vi "Rapid Read_5Ch.vi"(0 "Dig Cards":refnum<k15>[](array[refnum]), 2 "Pause?":bool, 5 "Motion Board ID":T1=1 min=1 max=32 step=1, 9 "rf points per line":i32, 11 "error in":errorcluster, 12 "lines per plane":i32, 13 "queue out":refnum<queue>) -> (1 "gain":dbl, 6 "Reverse?":bool, 10 "Dig Word Size":u16, 15 "error out":errorcluster)   [LabVIEW 2022 SP3]
uses:
  Motion Controllers/-MotionRoutines/MotionGlobals.vi
  <instrlib>/niScope/Acquire/Fetch/niScope Multi Fetch Binary 8.vi
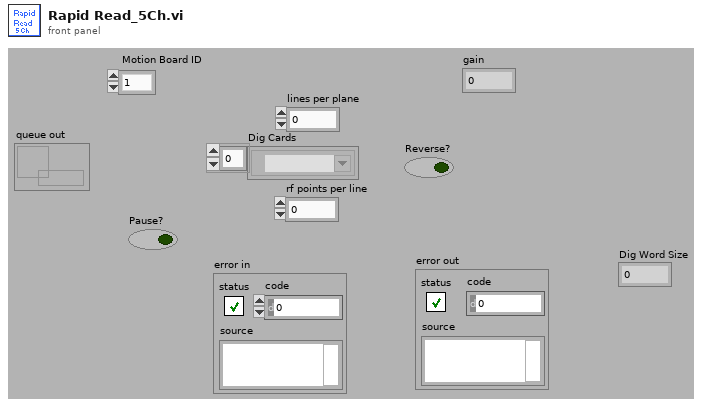
[diagram p1: front panel]
types:
  T1 = typedef "Board Id" = u8
  T2 = cluster{"Dig Cards[0]":refnum<k15>, "Dig Cards[1]":refnum<k15>, "Dig Cards[2]":refnum<k15>}
  T3 = typedef "Var" = u8
  T4 = cluster{"actualSamples":i32, "absoluteInitialX":dbl, "relativeInitialX":dbl, "xIncrement":dbl, "offset":dbl, "gain":dbl, "reserved1":dbl, "reserved2":dbl}[]
  T5 = cluster{"actualSamples":i32, "absoluteInitialX":dbl, "relativeInitialX":dbl, "xIncrement":dbl, "offset":dbl, "gain":dbl, "reserved1":dbl, "reserved2":dbl}
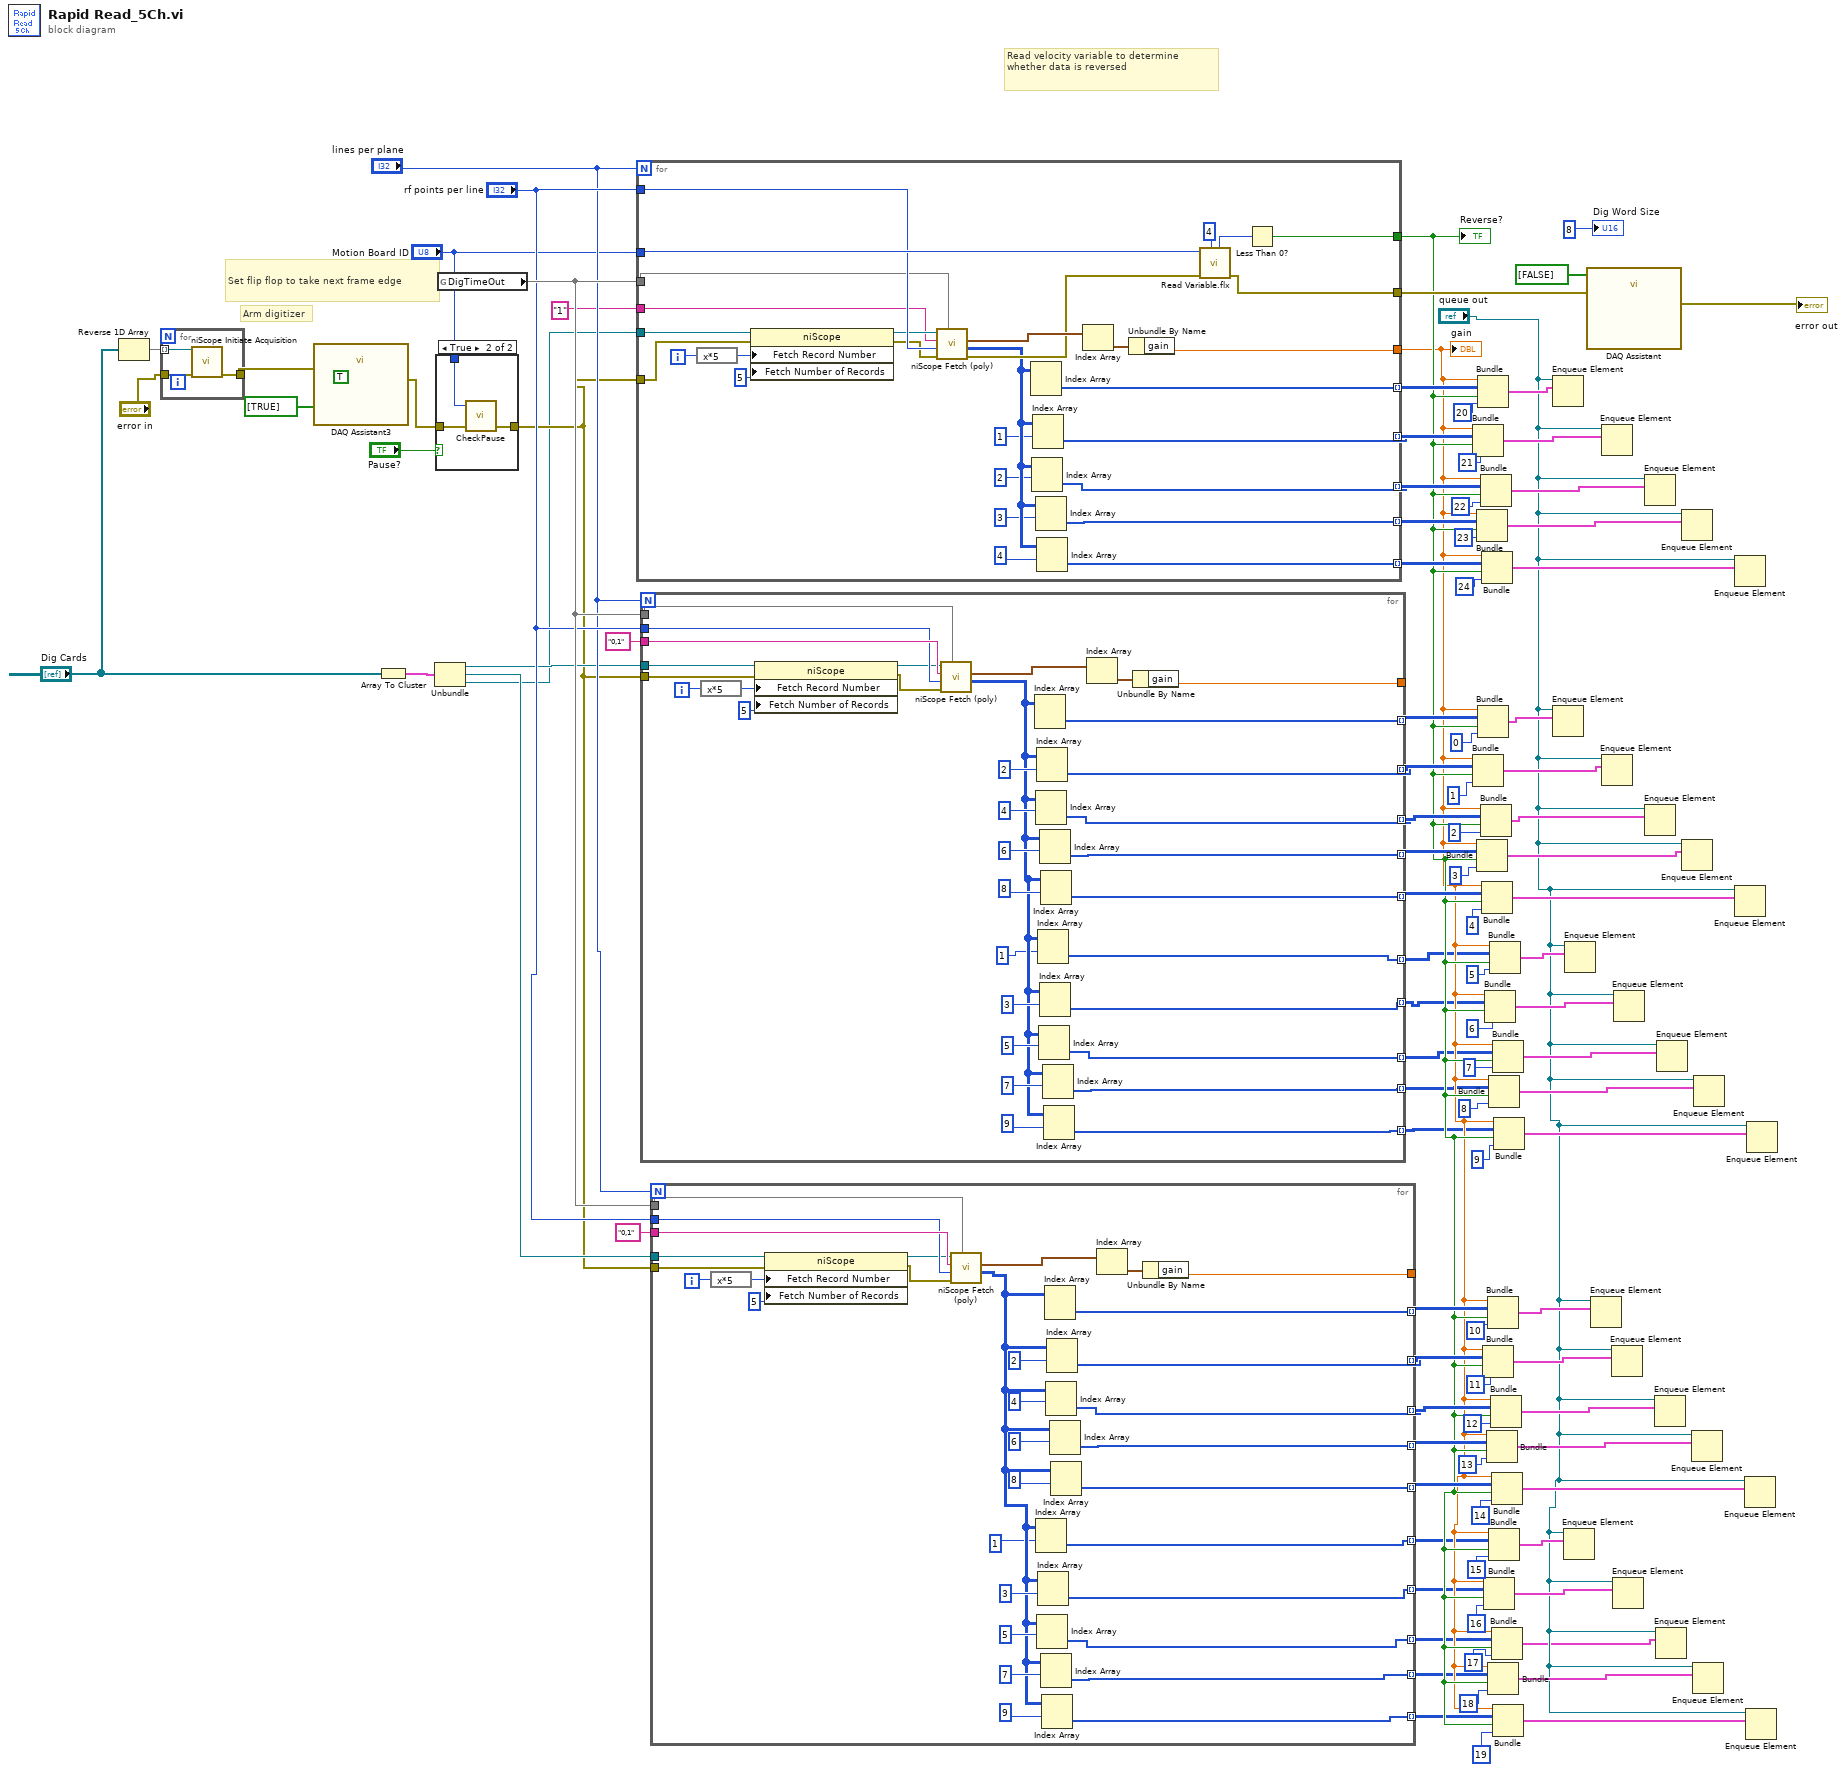
[diagram p0: block diagram]
diagram:
  (unwired) TRUE ("stop (T)")
  # "Set flip flop to take next frame edge"
  # "Arm digitizer"
  # "Read velocity variable to determine whether data is reversed"
  n1 = Reverse 1D Array(array="Dig Cards") -> (reversed array=w37:refnum<k15>[])
  n2 = for {
    tunnel: w37 -> [w104] mode=indexing
    tunnel: [w103] -> w36
    tunnel: "error in" -> [w102]
    n3 = call <instrlib>:"niScope Initiate Acquisition.vi"("instrument handle"=w104, "error in"=w102) -> ("error out"=w103:errorcluster)  [unwired: 1 in, 12 out]
  }
  n4 = call "DAQ Assistant3"("data"=bool[] [TRUE], "error in"=w36) -> ("error out"=w42:errorcluster)  [unwired: 2 in, 15 out]
  n5 = Array To Cluster(array="Dig Cards") -> (cluster=w97:T2)
  n6 = Unbundle(w97) -> ("Dig Cards[0]"=w44:refnum<k15>, "Dig Cards[1]"=w43:refnum<k15>, "Dig Cards[2]"=w35:refnum<k15>)
  n7 = case shown="True" "Pause?" {
    tunnel: w42 -> [w105 w108]
    tunnel: [w105 w107] -> w41
    tunnel: "Motion Board ID" -> [_ w106]
    frame False {
    }
    frame True {
      n8 = call "CheckPause.vi"("error in"=w108, "Motion Board ID"=w106) -> ("error out"=w107:errorcluster)  [unwired: 3 in]
    }
  }
  n9 = global read "MotionGlobals.vi" "DigTimeOut"() -> (w58)
  n10 = for {
    N: "lines per plane" -> [_]
    tunnel: "Motion Board ID" -> [w137]
    tunnel: "rf points per line" -> [w136]
    tunnel: w58 -> [w135]
    tunnel: w35 -> [w134]
    tunnel: w41 -> [w133]
    tunnel: "1" ("Channel") -> [w125]
    tunnel: [w119] -> w96 mode=indexing
    tunnel: [w118] -> w95 mode=indexing
    tunnel: [w117] -> w94 mode=indexing
    tunnel: [w116] -> w93 mode=indexing
    tunnel: [w115] -> w92 mode=indexing
    tunnel: [w111] -> w60
    tunnel: [w110] -> w59
    tunnel: [w109] -> w87
    i -> [w126]
    n11 = expression code="x*5"(w126) -> (w127:i32)
    n12 = property class="niScope"(reference=w134, error in=w133, "Fetch Record Number"=w127, "Fetch Number of Records"=5) -> (reference out=w132:refnum<k15>, error out=w131:errorcluster)
    n13 = call-poly <instrlib>:"niScope Fetch (poly).vi"("timeout"=w135, "error in"=w131, "numSamples"=w136, "channels"=w125, "instrument handle"=w132) -> ("error out"=w129:errorcluster, "wfm"=w124:i8[][], "wfm info"=w130:T4)  [unwired: 4 out]
    n14 = Index Array(array=w124) -> (element=w119:i8[])  [unwired: 2 in]
    n15 = Index Array(array=w124, index (row)=2) -> (element=w117:i8[])  [unwired: 1 in]
    n16 = Index Array(array=w124, index (row)=1) -> (element=w118:i8[])  [unwired: 1 in]
    n17 = Index Array(array=w124, index (row)=3) -> (element=w116:i8[])  [unwired: 1 in]
    n18 = Index Array(array=w124, index (row)=4) -> (element=w115:i8[])  [unwired: 1 in]
    n19 = Index Array(array=w130) -> (element=w112:T5)  [unwired: 1 in]
    n20 = Unbundle By Name(w112) -> ("gain"=w110:dbl)
    n21 = call <vilib>:"Read Variable.flx"("Var"=T3 4, "error in (no error)"=w129, "Board ID"=w137) -> ("error out"=w109:errorcluster, "Output"=w113:i32)  [unwired: 1 in, 4 out]
    n22 = Less Than 0?(x=w113) -> (x < 0?=w111:bool)
  }
  "Reverse?" <- w60
  "gain" <- w59
  n23 = for {
    N: "lines per plane" -> [_]
    tunnel: "rf points per line" -> [w150]
    tunnel: w58 -> [w148]
    tunnel: w44 -> [w170]
    tunnel: "0,1" ("Channel") -> [w165]
    tunnel: [w161] -> w85 mode=indexing
    tunnel: [w160] -> w84 mode=indexing
    tunnel: [w159] -> w83 mode=indexing
    tunnel: [w158] -> w82 mode=indexing
    tunnel: [w157] -> w81 mode=indexing
    tunnel: [w155] -> _
    tunnel: [w146] -> w55 mode=indexing
    tunnel: [w145] -> w54 mode=indexing
    tunnel: [w144] -> w53 mode=indexing
    tunnel: [w143] -> w52 mode=indexing
    tunnel: [w142] -> w51 mode=indexing
    tunnel: w41 -> [w141]
    i -> [w166]
    n24 = expression code="x*5"(w166) -> (w167:i32)
    n25 = property class="niScope"(reference=w170, error in=w141, "Fetch Record Number"=w167, "Fetch Number of Records"=5) -> (reference out=w149:refnum<k15>, error out=w147:errorcluster)
    n26 = call-poly <instrlib>:"niScope Fetch (poly).vi"("timeout"=w148, "error in"=w147, "numSamples"=w150, "channels"=w165, "instrument handle"=w149) -> ("wfm"=w139:i8[][], "wfm info"=w169:T4)  [unwired: 5 out]
    n27 = Index Array(array=w139) -> (element=w161:i8[])  [unwired: 2 in]
    n28 = Index Array(array=w139, index (row)=4) -> (element=w159:i8[])  [unwired: 1 in]
    n29 = Index Array(array=w139, index (row)=2) -> (element=w160:i8[])  [unwired: 1 in]
    n30 = Index Array(array=w139, index (row)=1) -> (element=w146:i8[])  [unwired: 1 in]
    n31 = Index Array(array=w139, index (row)=5) -> (element=w144:i8[])  [unwired: 1 in]
    n32 = Index Array(array=w139, index (row)=6) -> (element=w158:i8[])  [unwired: 1 in]
    n33 = Index Array(array=w139, index (row)=3) -> (element=w145:i8[])  [unwired: 1 in]
    n34 = Index Array(array=w139, index (row)=8) -> (element=w157:i8[])  [unwired: 1 in]
    n35 = Index Array(array=w139, index (row)=7) -> (element=w143:i8[])  [unwired: 1 in]
    n36 = Index Array(array=w139, index (row)=9) -> (element=w142:i8[])  [unwired: 1 in]
    n37 = Index Array(array=w169) -> (element=w156:T5)  [unwired: 1 in]
    n38 = Unbundle By Name(w156) -> ("gain"=w155:dbl)
  }
  n39 = for {
    N: "lines per plane" -> [_]
    tunnel: "rf points per line" -> [w182]
    tunnel: w58 -> [w181]
    tunnel: w43 -> [w203]
    tunnel: "0,1" ("Channel") -> [w198]
    tunnel: [w193] -> w69 mode=indexing
    tunnel: [w192] -> w68 mode=indexing
    tunnel: [w191] -> w67 mode=indexing
    tunnel: [w190] -> w66 mode=indexing
    tunnel: [w189] -> w65 mode=indexing
    tunnel: [w187] -> _
    tunnel: [w178] -> w50 mode=indexing
    tunnel: [w177] -> w49 mode=indexing
    tunnel: [w176] -> w48 mode=indexing
    tunnel: [w175] -> w47 mode=indexing
    tunnel: [w174] -> w46 mode=indexing
    tunnel: w41 -> [w173]
    i -> [w199]
    n40 = expression code="x*5"(w199) -> (w200:i32)
    n41 = property class="niScope"(reference=w203, error in=w173, "Fetch Record Number"=w200, "Fetch Number of Records"=5) -> (reference out=w180:refnum<k15>, error out=w179:errorcluster)
    n42 = call-poly <instrlib>:"niScope Fetch (poly).vi"("timeout"=w181, "error in"=w179, "numSamples"=w182, "channels"=w198, "instrument handle"=w180) -> ("wfm"=w172:i8[][], "wfm info"=w202:T4)  [unwired: 5 out]
    n43 = Index Array(array=w172, index (row)=1) -> (element=w178:i8[])  [unwired: 1 in]
    n44 = Index Array(array=w172, index (row)=5) -> (element=w176:i8[])  [unwired: 1 in]
    n45 = Index Array(array=w172, index (row)=3) -> (element=w177:i8[])  [unwired: 1 in]
    n46 = Index Array(array=w172, index (row)=7) -> (element=w175:i8[])  [unwired: 1 in]
    n47 = Index Array(array=w172, index (row)=9) -> (element=w174:i8[])  [unwired: 1 in]
    n48 = Index Array(array=w172) -> (element=w193:i8[])  [unwired: 2 in]
    n49 = Index Array(array=w172, index (row)=4) -> (element=w191:i8[])  [unwired: 1 in]
    n50 = Index Array(array=w172, index (row)=2) -> (element=w192:i8[])  [unwired: 1 in]
    n51 = Index Array(array=w172, index (row)=6) -> (element=w190:i8[])  [unwired: 1 in]
    n52 = Index Array(array=w172, index (row)=8) -> (element=w189:i8[])  [unwired: 1 in]
    n53 = Index Array(array=w202) -> (element=w188:T5)  [unwired: 1 in]
    n54 = Unbundle By Name(w188) -> ("gain"=w187:dbl)
  }
  n55 = Bundle("gain"=w59, "wfm"=w95, w60, 21) -> (w91:cluster{"gain":dbl, "wfm":i8[][], bool, i32})  [unwired: 1 in]
  n56 = Bundle("gain"=w59, "wfm"=w84, w60, 1) -> (w6:cluster{"gain":dbl, "wfm":i8[][], bool, i32})  [unwired: 1 in]
  n57 = Bundle("gain"=w59, "wfm"=w93, w60, 23) -> (w89:cluster{"gain":dbl, "wfm":i8[][], bool, i32})  [unwired: 1 in]
  n58 = Bundle("gain"=w59, "wfm"=w82, w60, 3) -> (w8:cluster{"gain":dbl, "wfm":i8[][], bool, i32})  [unwired: 1 in]
  n59 = Bundle("gain"=w59, "wfm"=w96, w60, 20) -> (w4:cluster{"gain":dbl, "wfm":i8[][], bool, i32})  [unwired: 1 in]
  n60 = Bundle("gain"=w59, "wfm"=w85, w60, 0) -> (w5:cluster{"gain":dbl, "wfm":i8[][], bool, i32})  [unwired: 1 in]
  n61 = Bundle("gain"=w59, "wfm"=w94, w60, 22) -> (w90:cluster{"gain":dbl, "wfm":i8[][], bool, i32})  [unwired: 1 in]
  n62 = Bundle("gain"=w59, "wfm"=w83, w60, 2) -> (w7:cluster{"gain":dbl, "wfm":i8[][], bool, i32})  [unwired: 1 in]
  n63 = Bundle("gain"=w59, "wfm"=w92, w60, 24) -> (w88:cluster{"gain":dbl, "wfm":i8[][], bool, i32})  [unwired: 1 in]
  n64 = Bundle("gain"=w59, "wfm"=w81, w60, 4) -> (w9:cluster{"gain":dbl, "wfm":i8[][], bool, i32})  [unwired: 1 in]
  n65 = Bundle("gain"=w59, "wfm"=w68, w60, 11) -> (w73:cluster{"gain":dbl, "wfm":i8[][], bool, i32})  [unwired: 1 in]
  n66 = Bundle("gain"=w59, "wfm"=w49, w60, 16) -> (w63:cluster{"gain":dbl, "wfm":i8[][], bool, i32})  [unwired: 1 in]
  n67 = Bundle("gain"=w59, "wfm"=w54, w60, 6) -> (w79:cluster{"gain":dbl, "wfm":i8[][], bool, i32})  [unwired: 1 in]
  n68 = Bundle("gain"=w59, "wfm"=w66, w60, 13) -> (w71:cluster{"gain":dbl, "wfm":i8[][], bool, i32})  [unwired: 1 in]
  n69 = Bundle("gain"=w59, "wfm"=w69, w60, 10) -> (w74:cluster{"gain":dbl, "wfm":i8[][], bool, i32})  [unwired: 1 in]
  n70 = Bundle("gain"=w59, "wfm"=w47, w60, 18) -> (w62:cluster{"gain":dbl, "wfm":i8[][], bool, i32})  [unwired: 1 in]
  n71 = Bundle("gain"=w59, "wfm"=w52, w60, 8) -> (w77:cluster{"gain":dbl, "wfm":i8[][], bool, i32})  [unwired: 1 in]
  n72 = Bundle("gain"=w59, "wfm"=w50, w60, 15) -> (w64:cluster{"gain":dbl, "wfm":i8[][], bool, i32})  [unwired: 1 in]
  n73 = Bundle("gain"=w59, "wfm"=w55, w60, 5) -> (w80:cluster{"gain":dbl, "wfm":i8[][], bool, i32})  [unwired: 1 in]
  n74 = Bundle("gain"=w59, "wfm"=w67, w60, 12) -> (w72:cluster{"gain":dbl, "wfm":i8[][], bool, i32})  [unwired: 1 in]
  n75 = Bundle("gain"=w59, "wfm"=w65, w60, 14) -> (w70:cluster{"gain":dbl, "wfm":i8[][], bool, i32})  [unwired: 1 in]
  n76 = Bundle("gain"=w59, "wfm"=w48, w60, 17) -> (w2:cluster{"gain":dbl, "wfm":i8[][], bool, i32})  [unwired: 1 in]
  n77 = Bundle("gain"=w59, "wfm"=w53, w60, 7) -> (w78:cluster{"gain":dbl, "wfm":i8[][], bool, i32})  [unwired: 1 in]
  n78 = Bundle("gain"=w59, "wfm"=w46, w60, 19) -> (w61:cluster{"gain":dbl, "wfm":i8[][], bool, i32})  [unwired: 1 in]
  n79 = Bundle("gain"=w59, "wfm"=w51, w60, 9) -> (w76:cluster{"gain":dbl, "wfm":i8[][], bool, i32})  [unwired: 1 in]
  n80 = Enqueue Element(queue="queue out", element=w4) -> ()  [unwired: 2 in, 3 out]
  n81 = Enqueue Element(queue="queue out", element=w5) -> ()  [unwired: 2 in, 3 out]
  n82 = Enqueue Element(queue="queue out", element=w64) -> ()  [unwired: 2 in, 3 out]
  n83 = Enqueue Element(queue="queue out", element=w80) -> ()  [unwired: 2 in, 3 out]
  n84 = call "DAQ Assistant"("data"=bool[] [FALSE], "error in"=w87) -> ("error out"=→"error out":errorcluster)  [unwired: 2 in, 15 out]
  n85 = Enqueue Element(queue="queue out", element=w74) -> ()  [unwired: 2 in, 3 out]
  n86 = Enqueue Element(queue="queue out", element=w91) -> ()  [unwired: 2 in, 3 out]
  n87 = Enqueue Element(queue="queue out", element=w6) -> ()  [unwired: 2 in, 3 out]
  n88 = Enqueue Element(queue="queue out", element=w73) -> ()  [unwired: 2 in, 3 out]
  n89 = Enqueue Element(queue="queue out", element=w63) -> ()  [unwired: 2 in, 3 out]
  n90 = Enqueue Element(queue="queue out", element=w79) -> ()  [unwired: 2 in, 3 out]
  n91 = Enqueue Element(queue="queue out", element=w90) -> ()  [unwired: 2 in, 3 out]
  n92 = Enqueue Element(queue="queue out", element=w7) -> ()  [unwired: 2 in, 3 out]
  n93 = Enqueue Element(queue="queue out", element=w72) -> ()  [unwired: 2 in, 3 out]
  n94 = Enqueue Element(queue="queue out", element=w2) -> ()  [unwired: 2 in, 3 out]
  n95 = Enqueue Element(queue="queue out", element=w78) -> ()  [unwired: 2 in, 3 out]
  n96 = Enqueue Element(queue="queue out", element=w89) -> ()  [unwired: 2 in, 3 out]
  n97 = Enqueue Element(queue="queue out", element=w8) -> ()  [unwired: 2 in, 3 out]
  n98 = Enqueue Element(queue="queue out", element=w71) -> ()  [unwired: 2 in, 3 out]
  n99 = Enqueue Element(queue="queue out", element=w62) -> ()  [unwired: 2 in, 3 out]
  n100 = Enqueue Element(queue="queue out", element=w77) -> ()  [unwired: 2 in, 3 out]
  n101 = Enqueue Element(queue="queue out", element=w88) -> ()  [unwired: 2 in, 3 out]
  n102 = Enqueue Element(queue="queue out", element=w9) -> ()  [unwired: 2 in, 3 out]
  n103 = Enqueue Element(queue="queue out", element=w70) -> ()  [unwired: 2 in, 3 out]
  n104 = Enqueue Element(queue="queue out", element=w61) -> ()  [unwired: 2 in, 3 out]
  n105 = Enqueue Element(queue="queue out", element=w76) -> ()  [unwired: 2 in, 3 out]
  "Dig Word Size" <- 8
